vi "Embdata_Creator.vi"(0 "Pre File":string, 1 "Post File":string, 2 "root path":path, 3 "error in (no error)":errorcluster) -> (7 "Pre-EBD Data (U8)":u8[](array[numeric]), 8 "Post-EBD Data (U8)":u8[](array[numeric]), 9 "EBD Config":T1, 10 "error out":errorcluster)   [LabVIEW 2020]
uses:
  ctl/Image_EBD_Config.ctl
panel:
  out "concatenated string":string
  out "standard error":string
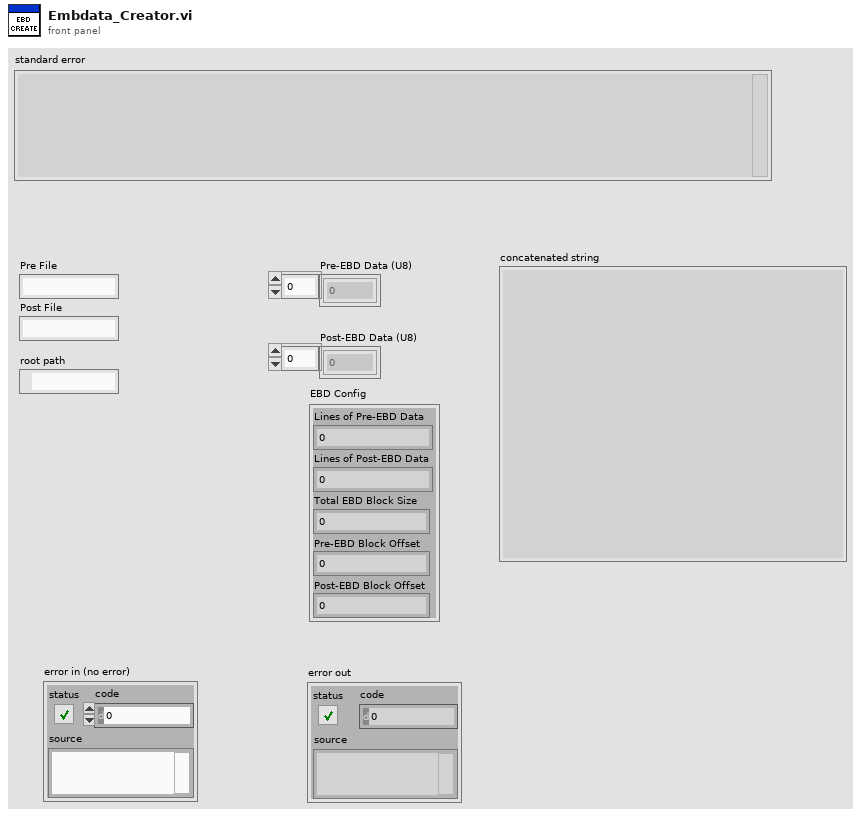
[diagram p1: front panel]
types:
  T1 = typedef "Image_EBD_Config.ctl" = cluster{"Lines of Pre-EBD Data":u16, "Lines of Post-EBD Data":u16, "Total EBD Block Size":u32, "Pre-EBD Block Offset ":u32, "Post-EBD Block Offset ":u32}
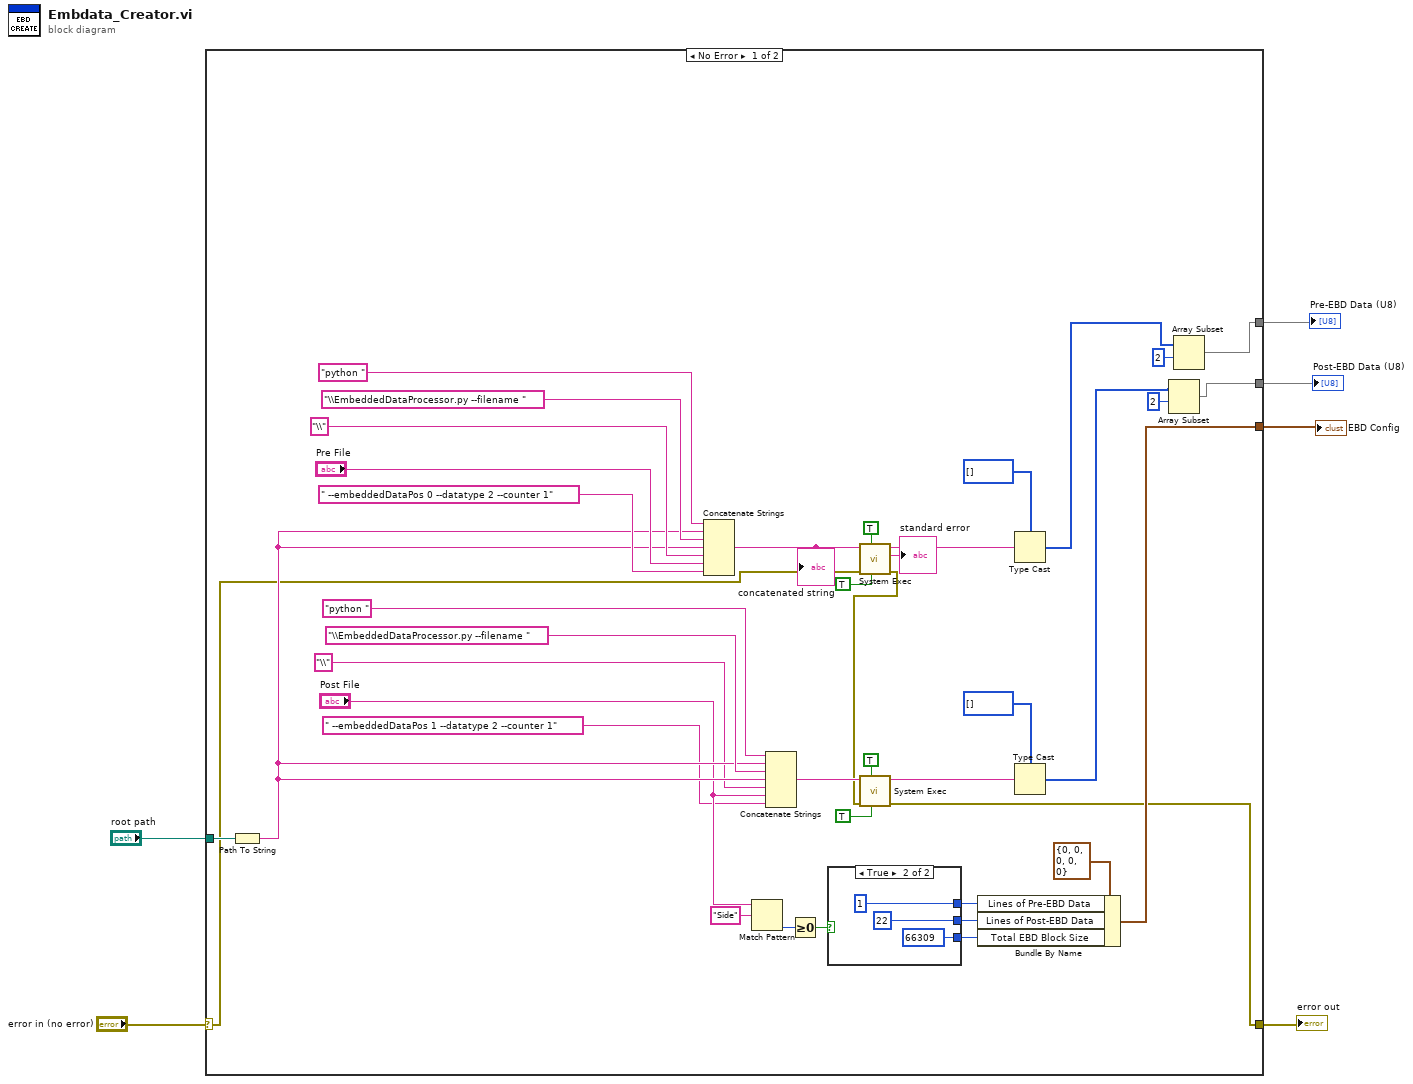
[diagram p0: block diagram]
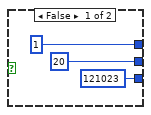
[diagram p2: hidden frame]
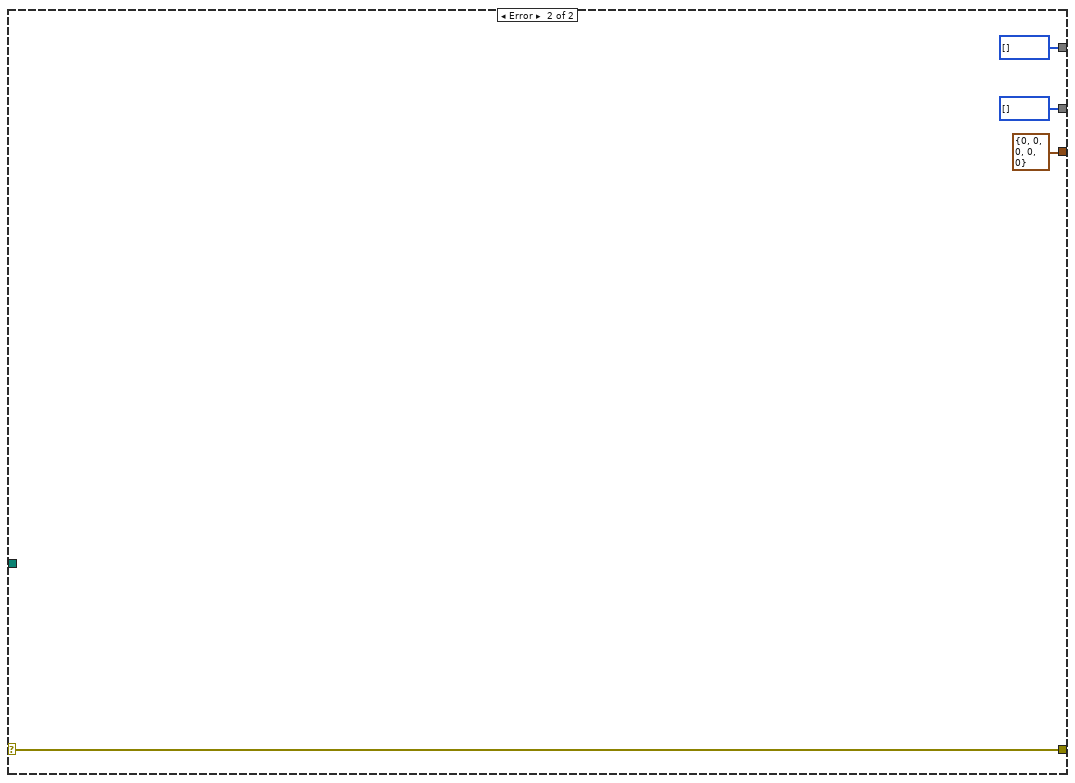
[diagram p3: hidden frame]
diagram:
  n1 = case shown="No Error" "error in (no error)" {
    selector: "error in (no error)" -> [w15 w56]
    tunnel: [w13 w56] -> w5
    tunnel: [w11 u8[] [] ("Pre-EBD Data (U8)")] -> w4
    tunnel: [w9 u8[] [] ("Pre-EBD Data (U8)")] -> w3
    tunnel: [w36 T1 {"Lines of Pre-EBD Data"=0, "Lines of Post-EBD Data"=0, "Total EBD Block Size"=0, "Pre-EBD Block Offset "=0, "Post-EBD Block Offset "=0} ("EBD Config")] -> w2
    tunnel: "root path" -> [w31 _]
    frame No Error {
      n2 = Path To String(path=w31) -> (string=w22:string)
      n3 = Concatenate Strings("python " ("command line"), w22, "\\EmbeddedDataProcessor.py --filename " ("string"), w22, "\\" ("string"), "Pre File", " --embeddedDataPos 0 --datatype 2 --counter 1" ("command line")) -> (w25:string)
      "concatenated string" <- w25
      n4 = Match Pattern(string="Post File", regular expression="Side") -> (offset past match=w38:i32)  [unwired: 1 in, 3 out]
      n5 = Concatenate Strings("python " ("command line"), w22, "\\EmbeddedDataProcessor.py --filename " ("string"), w22, "\\" ("string"), "Post File", " --embeddedDataPos 1 --datatype 2 --counter 1" ("command line")) -> (w41:string)
      n6 = Greater Or Equal To 0?(x=w38) -> (x >= 0?=w35:bool)
      n7 = case shown="True" w35 {
        tunnel: [u16 1 ("Lines of Pre-EBD Data") u16 1 ("Lines of Pre-EBD Data")] -> w34
        tunnel: [u16 20 ("Lines of Post-EBD Data") u16 22 ("Lines of Post-EBD Data")] -> w33
        tunnel: [u32 121023 ("Total EBD Block Size") u32 66309 ("Total EBD Block Size")] -> w32
        frame False {
        }
        frame True {
        }
      }
      n8 = call <vilib>:"System Exec.vi"("run minimized? (F)"=TRUE, "wait until completion? (T)"=TRUE, "error in (no error)"=w15, "command line"=w25) -> ("error out"=w14:errorcluster, "standard error"=→"standard error":string, "standard output"=w44:string)  [unwired: 4 in, 1 out]
      n9 = call <vilib>:"System Exec.vi"("run minimized? (F)"=TRUE, "wait until completion? (T)"=TRUE, "error in (no error)"=w14, "command line"=w41) -> ("error out"=w13:errorcluster, "standard output"=w40:string)  [unwired: 4 in, 2 out]
      n10 = Bundle By Name(cluster=T1 {"Lines of Pre-EBD Data"=0, "Lines of Post-EBD Data"=0, "Total EBD Block Size"=0, "Pre-EBD Block Offset "=0, "Post-EBD Block Offset "=0} ("EBD Config"), "Lines of Pre-EBD Data"=w34, "Lines of Post-EBD Data"=w33, "Total EBD Block Size"=w32) -> (w36:T1)
      n11 = Type Cast(type=u8[] [], x=w44) -> (*(type *) &x=w12:u8[])
      n12 = Type Cast(type=u8[] [], x=w40) -> (*(type *) &x=w10:u8[])
      n13 = Array Subset(array=w10, index=2) -> (w9:u8[])  [unwired: 1 in]
      n14 = Array Subset(array=w12, index=2) -> (w11:u8[])  [unwired: 1 in]
    }
    frame Error {
    }
  }
  "error out" <- w5
  "EBD Config" <- w2
  "Pre-EBD Data (U8)" <- w4
  "Post-EBD Data (U8)" <- w3
